vi "Configure Real Time Power.vi"(7 "Total Noise Power (0)":dbl, 8 "error in (no error)":errorcluster, 9 "Carrier Power (0)":dbl, 10 "Power Control Mode (0: Total)":i32(ring) items=["Total", "Carrier", "Noise"], 11 "VISA resource name":refnum<visa-resource-name>) -> (0 "error out":errorcluster, 3 "VISA resource name out":refnum<visa-resource-name>)   [LabVIEW 2014, in "Agilent PSG MXG Series.lvlib"]
doc: "Configure real time power settings.\n\n<B>Notes:</B>\n(1) This VI is valid only in N5172B and N5182B that install <B>Option 431</B> or <B>Option 403</B>."
uses:
  Agilent PSG MXG Series.lvlib
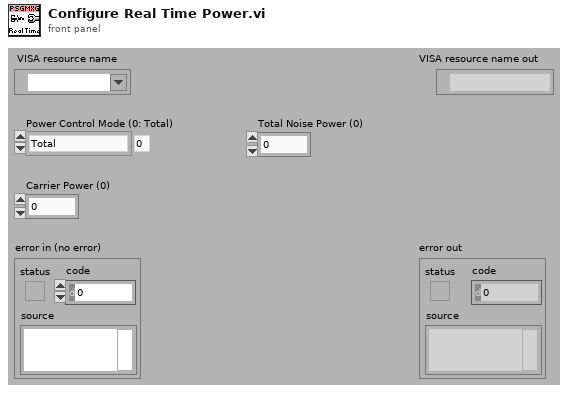
[diagram p1: front panel]
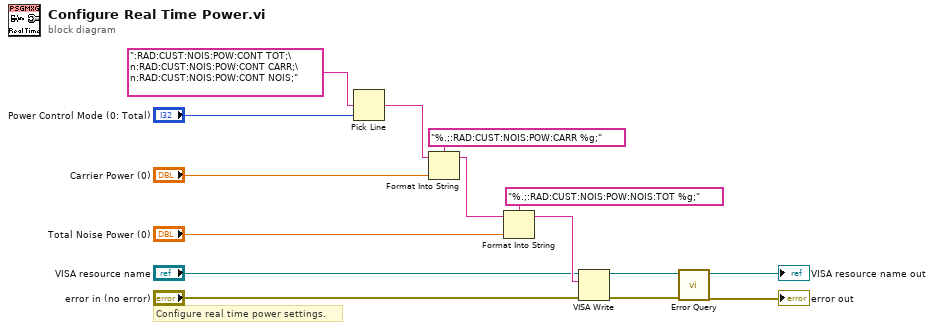
[diagram p0: block diagram]
diagram:
  # "Configure real time power settings."
  n1 = Pick Line(multi-line string=":RAD:CUST:NOIS:POW:CONT TOT;\n:RAD:CUST:NOIS:POW:CONT CARR;\n:RAD:CUST:NOIS:POW:CONT NOIS;", line index="Power Control Mode (0: Total)") -> (output string=w13:string)  [unwired: 1 out]
  n2 = Format Into String(format string="%.;:RAD:CUST:NOIS:POW:CARR %g;", initial string=w13, "Carrier Power (0)") -> (resulting string=w10:string)  [unwired: 1 in, 1 out]
  n3 = Format Into String(format string="%.;:RAD:CUST:NOIS:POW:NOIS:TOT %g;", initial string=w10, "Total Noise Power (0)") -> (resulting string=w7:string)  [unwired: 1 in, 1 out]
  n4 = VISA Write(VISA resource name="VISA resource name", write buffer=w7, error in (no error)="error in (no error)") -> (VISA resource name out=w4:refnum<visa-resource-name>, error out=w3:errorcluster)  [unwired: 1 out]
  n5 = call "Error Query.vi"("error in (no error)"=w3, "VISA resource name"=w4) -> ("error out"=→"error out":errorcluster, "VISA resource name out"=→"VISA resource name out":refnum<visa-resource-name>)  [unwired: 8 out]
